vi "Set simulated or real mode.vi"(8 "error in (no error)":errorcluster, 11 "Channel in":refnum<class "Channel.lvclass">) -> (0 "error out":errorcluster, 3 "Channel out":refnum<class "Channel.lvclass">)   [LabVIEW 2018, in "Channel.lvclass"]
doc: "Choose between the simulated or real camera class"
uses:
  Channel.lvclass
  CCDCamera/Real Camera.lvclass
  C:/Users/Denis/Desktop/S4CCS/S4CCS/Simulated_CCD_Camera/Simulated Camera.lvclass
  Channel.lvclass/Channel.ctl
panel:
  in  "CCDCamera.lvclass":refnum<class "Real Camera.lvclass">
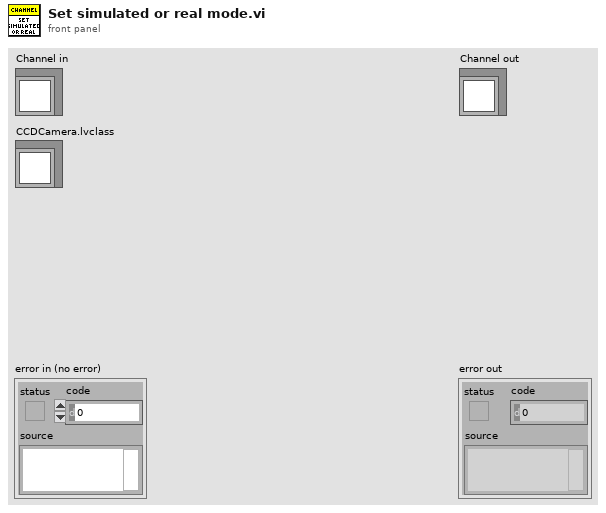
[diagram p1: front panel]
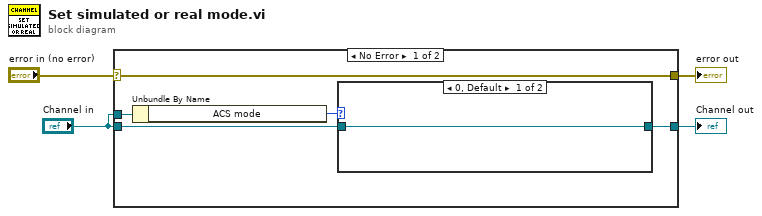
[diagram p0: block diagram]
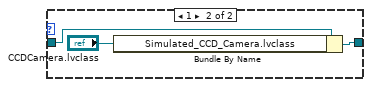
[diagram p2: hidden frame]
diagram:
  n1 = case shown="No Error" "error in (no error)" {
    selector: "error in (no error)" -> [w7 w15]
    tunnel: [w7 w15] -> w3
    tunnel: [w5 w14] -> w2
    tunnel: "Channel in" -> [w8 w14]
    tunnel: "Channel in" -> [w6 _]
    frame No Error {
      n2 = Unbundle By Name(w8) -> ("ACS mode"=w9:u16)
      n3 = case shown="0, Default" w9 {
        tunnel: w6 -> [w10 w13]
        tunnel: [w10 w11] -> w5
        frame 0, Default {
        }
        frame 1 {
          n4 = Bundle By Name(cluster=w13, "Simulated_CCD_Camera.lvclass"="CCDCamera.lvclass") -> (w11:refnum<class "Channel.lvclass">)
        }
      }
    }
    frame Error {
    }
  }
  "error out" <- w3
  "Channel out" <- w2
